vi "main.vi"() -> ()   [LabVIEW 2021]
uses:
  src/Material Theme/Material Theme.lvclass
panel:
  out "error out":errorcluster
  in  "save?":bool=TRUE
  out "theme":path
  in  "Theme Style":u16(ring) items=["Light", "Light Medium Contrast", "Light High Contrast", "Dark", "Dark Medium Contrast", "Dark High Contrast"]
  in  "File Path (theme)":path
  in  "filled--text--rectangular":bool
  in  "tonal--icons--rounded":bool
  in  "outline--text--rectangular":bool
  in  "FAB Button":bool
  # "control UI role = Primary"
  # "control UI role = Primary"
  # "Decoration--Surface Container Low"
  # "control UI role = Tertiary"
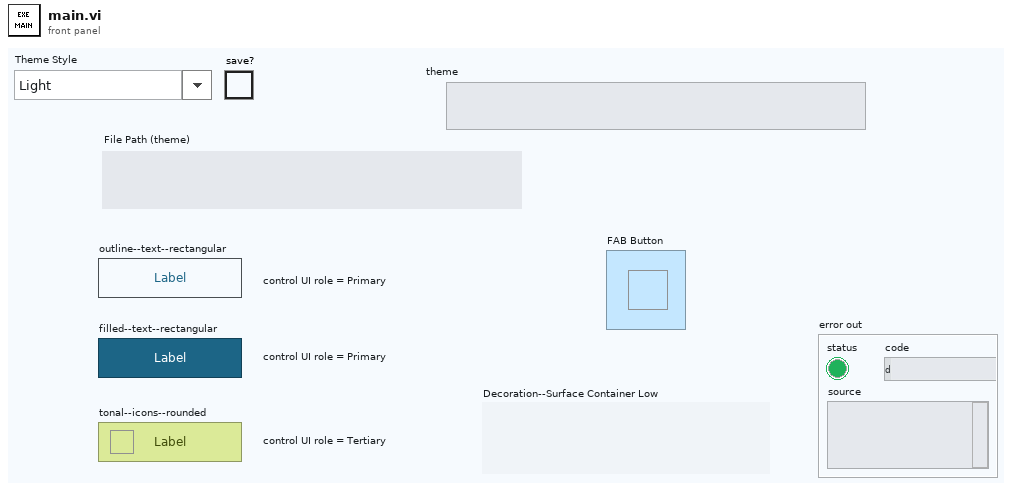
[diagram p1: front panel]
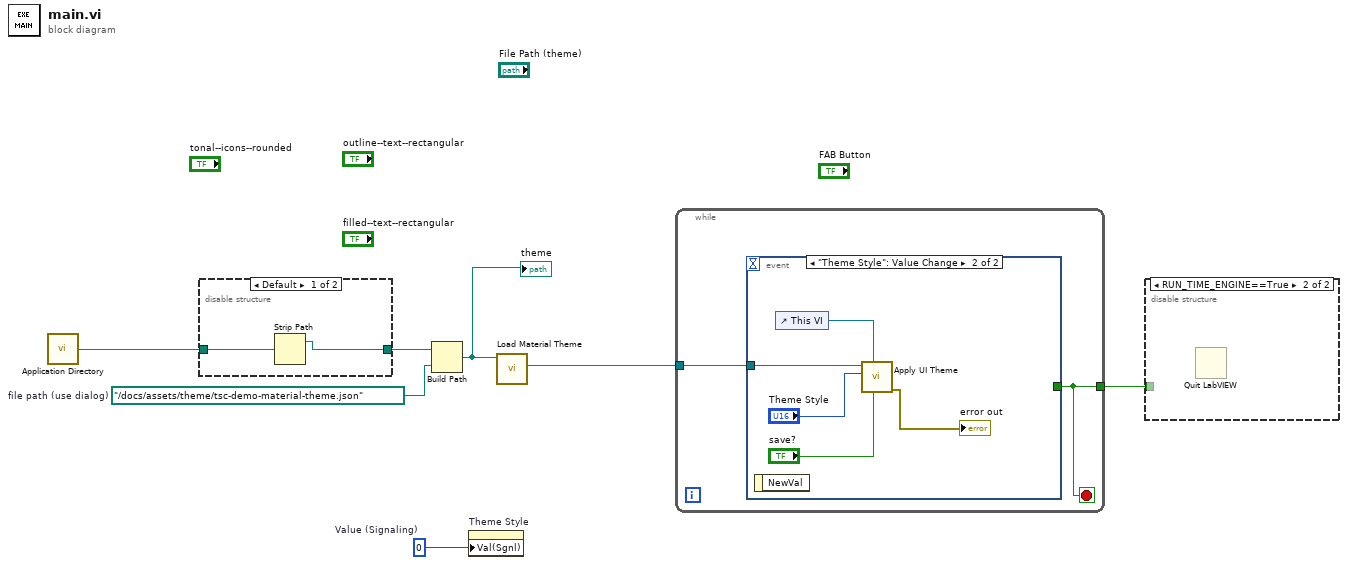
[diagram p0: block diagram]
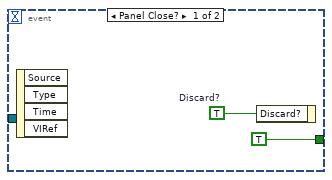
[diagram p4: hidden frame]
diagram:
  w1 = u16 0  # Value (Signaling)
  w6 = path "../docs/assets/theme/tsc-demo-material-theme.json"  # file path (use dialog)
  n1 = call <vilib>:"Application Directory.vi"() -> ("Application Directory"=w5:path)
  n2 = disable-structure shown="Default" {
    disable-tunnel: w5 -> [w9 w10]
    disable-tunnel: [w8 w10] -> w4
    frame condition #0 (active) {
      n3 = Strip Path(path=w9) -> (stripped path=w8:path)  [unwired: 1 out]
    }
    frame condition #1 {
    }
  }
  n4 = Build Path(base path=w4, name or relative path=w6) -> (appended path=w3:path)
  "theme" <- w3
  n5 = property on="Theme Style" class="Ring (strict)"("Val(Sgnl)"=w1) -> ()  [unwired: 2 in, 2 out]
  n6 = call "Load Material Theme.vi"("file path"=w3) -> ("Theme"=w2:refnum<class "Material Theme.lvclass">)  [unwired: 8 in, 2 out]
  n7 = while {
    tunnel: [w12] -> w7
    tunnel: w2 -> [w11]
    stop <- w12 stop-if-true
    n8 = event shown="[1] \"Theme Style\": Value Change" {
      selector: _ -> [_ _]
      dyn-events: _ -> [_ _]
      timeout: _ -> [_ _]
      tunnel: [TRUE _] -> w12
      tunnel: w11 -> [_ w19]
      event Panel Close? {
        w14 = TRUE  # Discard?
        n9 = event-data() -> ()  [unwired: 1 in, 4 out]
        n10 = event-data("Discard?"=w14) -> ()  [unwired: 1 in, 1 out]
      }
      event "Theme Style": Value Change {
        n11 = event-data() -> ()  [unwired: 1 in, 1 out]
        n12 = control-ref of="This VI"() -> (w18:refnum<vi>)
        n13 = call "Apply UI Theme.vi"("save?"="save?", "VI Refnum"=w18, "Theme Mode"="Theme Style", "Material Theme in"=w19) -> ("error out"=→"error out":errorcluster)  [unwired: 6 in, 1 out]
      }
    }
  }
  n14 = disable-structure shown="RUN_TIME_ENGINE==True" {
    disable-tunnel: w7 -> [_ _]
    frame condition #0 (active) {
    }
    frame condition #1 {
      n15 = Quit LabVIEW() -> ()  [unwired: 1 in]
    }
  }
